vi "Test.vi"() -> ()   [LabVIEW 2014, in "SetUp VIs.lvlib" / "Instrument Finder.lvclass"]
uses:
  Instrument Finder.lvclass
  <vilib>/ActorFramework/Message Enqueuer/Message Enqueuer.lvclass/Message Enqueuer.ctl
  <vilib>/ActorFramework/Message Enqueuer/Enqueue.vi
  <vilib>/ActorFramework/Message Priority Queue/Priority Enqueue.vi
  <vilib>/ActorFramework/Stop Msg/Stop Msg.lvclass
  <vilib>/ActorFramework/Actor/Actor.lvclass
panel:
  out "error out":errorcluster
  in  "Stop Button":bool
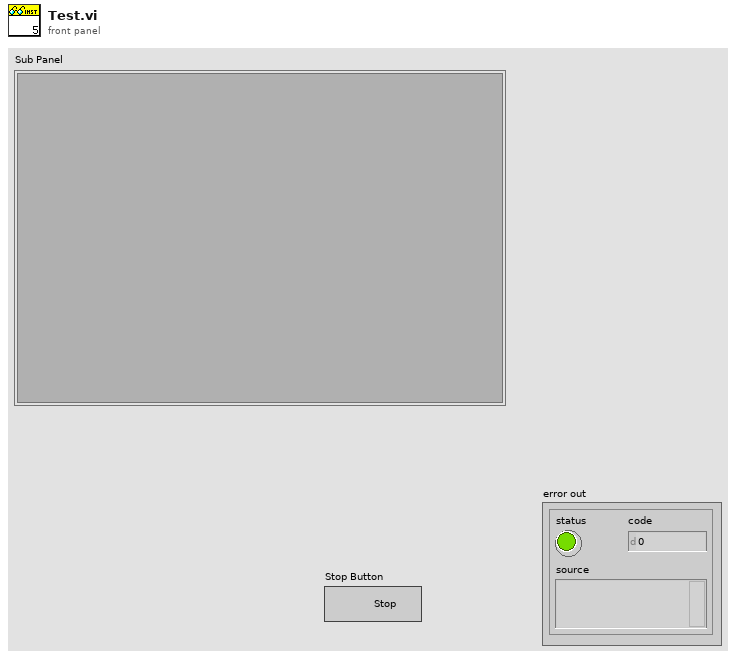
[diagram p1: front panel]
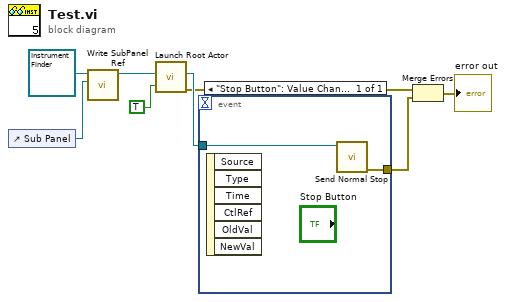
[diagram p0: block diagram]
diagram:
  n1 = control-ref of="Sub Panel"() -> (w1:refnum<vi>)
  n2 = call-dynamic "Write SubPanel Ref.vi"("SubPanel Ref"=w1, "Subpanel Inserter in"=refnum<class "Instrument Finder.lvclass"> refnum ("SetUp VIs.lvlib:Instrument Finder.lvclass")) -> ("Subpanel Inserter out"=w2:refnum<class "Instrument Finder.lvclass">)  [unwired: 8 in, 1 out]
  n3 = call <vilib>:"Launch Root Actor.vi"("Open Actor Core front panel? (F)"=TRUE, "Actor"=w2) -> ("error out"=w5:errorcluster, "Actor's Enqueuer"=w7:refnum<class "Message Enqueuer.lvclass">)  [unwired: 8 in]
  n4 = event shown="[0] \"Stop Button\": Value Change" {
    selector: _ -> [_]
    dyn-events: _ -> [_]
    timeout: _ -> [_]
    tunnel: w7 -> [w10]
    tunnel: [w9] -> w6
    event "Stop Button": Value Change {
      n5 = event-data() -> ()  [unwired: 1 in, 6 out]
      n6 = call <vilib>:"Send Normal Stop.vi"("Message Enqueuer"=w10) -> ("error out"=w9:errorcluster)  [unwired: 10 in]
    }
  }
  n7 = Merge Errors(w5, w6) -> (→"error out":errorcluster)
